vi "Get image percentile.vi"(7 "Percentile (95%)":dbl=95.0, 8 "error in (no error)":errorcluster, 11 "Image":T1) -> (0 "error out":errorcluster, 3 "percentile":dbl)   [LabVIEW 2009]
uses:
  <vilib>/vision/Image Controls.llb/IMAQ Image.ctl
  <vilib>/gmath/statdist.llb/st_Percentiles (scalar).vi
  <vilib>/gmath/NI_Gmath.lvlib
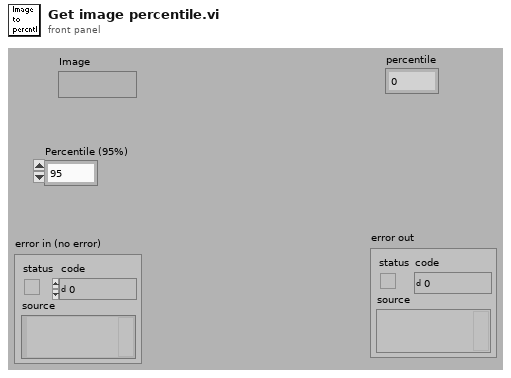
[diagram p1: front panel]
types:
  T1 = typedef "IMAQ Image.ctl" = refnum<image>
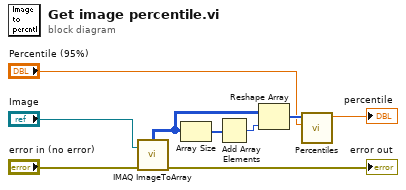
[diagram p0: block diagram]
diagram:
  n1 = call "IMAQ ImageToArray"("error in (no error)"="error in (no error)", "Image"="Image") -> ("error out"=→"error out":errorcluster, "Image Pixels (U8)"=w9:u8[][])  [unwired: 1 in, 4 out]
  n2 = Array Size(array=w9) -> (size(s)=w8:i32[])
  n3 = Add Array Elements(numeric array=w8) -> (sum=w7:i32)
  n4 = Reshape Array(w9, w7) -> (w6:u8[])
  n5 = call-poly <vilib>:"Percentiles.vi"("p"="Percentile (95%)", "x array"=w6) -> ("percentile"=→"percentile":dbl)  [unwired: 9 out]
